vi "Handle Collision.vi"(8 "Cluster":T1, 9 "Column":i32, 10 "Row":i32, 11 "Temp DVR":refnum<data-value>) -> (3 "Temp DVR":refnum<data-value>)   [LabVIEW 2015, in "SB SubVIs.lvlib"]
uses:
  SB SubVIs.lvlib
  Type Defs/Square Cluster.ctl
  Square/Square.lvclass
  Globals.vi
  Type Defs/SB Type Defs.lvlib
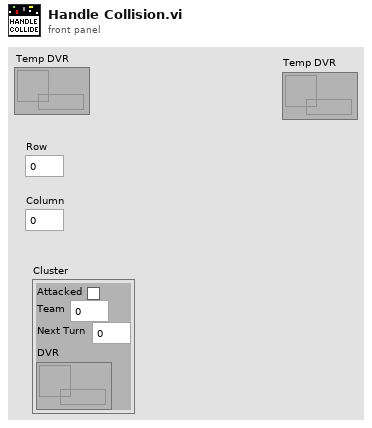
[diagram p1: front panel]
types:
  T1 = typedef "SB Type Defs.lvlib/Square Cluster.ctl" = cluster{"Attacked":bool, "Team":i32, "Next Turn":i32, "DVR":refnum<data-value>}
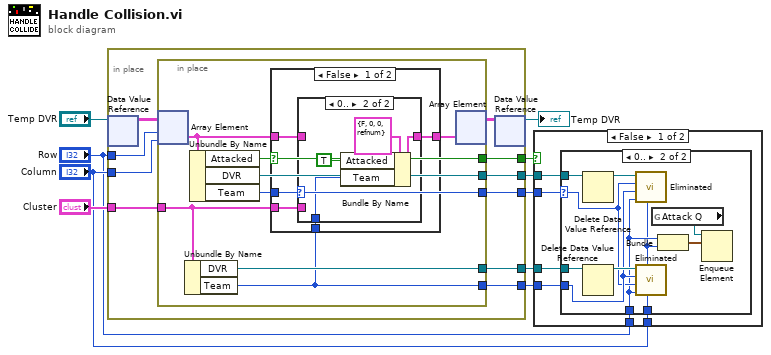
[diagram p0: block diagram]
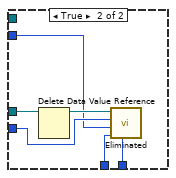
[diagram p3: hidden frame]
diagram:
  n1 = in-place {
    in-place-border: "Row" -> [w13]
    in-place-border: "Column" -> [w12]
    in-place-border: "Cluster" -> [w18]
    in-place-border: [w17] -> w7
    in-place-border: [w16] -> w6
    in-place-border: [w15] -> w5
    in-place-border: [w14] -> w4
    in-place-border: [w11] -> w3
    n2 = in-place-dvr #1("Temp DVR") -> (w20:T1[][])  [unwired: 1 out]
    n3 = in-place {
      in-place-border: w18 -> [w26]
      in-place-border: [w25] -> w17
      in-place-border: [w24] -> w16
      in-place-border: [w23] -> w15
      in-place-border: [w22] -> w14
      in-place-border: [w21] -> w11
      n4 = in-place-array #2(w20, w13, w12) -> (w27:T1)
      n5 = Unbundle By Name(w26) -> ("DVR"=w22:refnum<data-value>, "Team"=w21:i32)
      n6 = Unbundle By Name(w27) -> ("Attacked"=w25:bool, "DVR"=w24:refnum<data-value>, "Team"=w23:i32)
      n7 = case shown="False" w25 {
        tunnel: [w31 w39] -> w28
        tunnel: w27 -> [w32 w39]
        tunnel: w23 -> [w33 _]
        tunnel: w26 -> [w30 _]
        tunnel: w21 -> [w29 _]
        frame False {
          n8 = case shown="0.." w33 {
            tunnel: w32 -> [_ _]
            tunnel: [w34 w37] -> w31
            tunnel: w30 -> [w34 _]
            tunnel: w29 -> [_ w35]
            frame ..-1 {
            }
            frame 0.. {
              n9 = Bundle By Name(cluster=T1 {"Attacked"=FALSE, "Team"=0, "Next Turn"=0, "DVR"=refnum} ("Cluster"), "Attacked"=TRUE, "Team"=w35) -> (w37:T1)
            }
          }
        }
        frame True {
        }
      }
      n10 = in-place-array #2(w28) -> (w19:T1[][])  [unwired: 2 out]
    }
    n11 = in-place-dvr #1(w19) -> (→"Temp DVR":refnum<data-value>)  [unwired: 1 out]
  }
  n12 = case shown="False" w7 {
    tunnel: w4 -> [w43 w61]
    tunnel: w6 -> [w45 _]
    tunnel: w5 -> [w44 w58]
    tunnel: w3 -> [w42 w59]
    tunnel: "Column" -> [w41 w57]
    tunnel: "Row" -> [w40 w56]
    frame False {
      n13 = case shown="0.." w44 {
        selector: w44 -> [_ w50]
        tunnel: w43 -> [_ w54]
        tunnel: w45 -> [_ w55]
        tunnel: w42 -> [_ w51]
        tunnel: w41 -> [_ w46]
        tunnel: w40 -> [_ w47]
        frame ..-1 {
        }
        frame 0.. {
          n14 = Delete Data Value Reference(data value reference=w55) -> (data value=w52:refnum<class "Square.lvclass">)  [unwired: 1 in, 1 out]
          n15 = Delete Data Value Reference(data value reference=w54) -> (data value=w53:refnum<class "Square.lvclass">)  [unwired: 1 in, 1 out]
          n16 = call-dynamic "Eliminated.vi"("Column"=w46, "Row"=w47, "Killer"=w51, "Team"=w50, "Square in"=w52) -> ()  [unwired: 6 in, 1 out]
          n17 = call-dynamic "Eliminated.vi"("Column"=w46, "Row"=w47, "Killer"=w50, "Team"=w51, "Square in"=w53) -> ()  [unwired: 6 in, 1 out]
          n18 = global read "Globals.vi" "Attack Q"() -> (w48:refnum<queue>)
          n19 = Bundle("Row"=w47, "Column"=w46) -> (w49:cluster{"Row":i32, "Column":i32})  [unwired: 1 in]
          n20 = Enqueue Element(queue=w48, element=w49) -> ()  [unwired: 2 in, 3 out]
        }
      }
    }
    frame True {
      n21 = Delete Data Value Reference(data value reference=w61) -> (data value=w60:refnum<class "Square.lvclass">)  [unwired: 1 in, 1 out]
      n22 = call-dynamic "Eliminated.vi"("Column"=w57, "Row"=w56, "Killer"=w58, "Team"=w59, "Square in"=w60) -> ()  [unwired: 6 in, 1 out]
    }
  }
